vi "Get New Index.vi"(10 "last index":i32, 11 "control index":i32) -> (3 "new index":i32)   [LabVIEW 2015, in "LVJSON.lvlib" / "Index JSON Array.xnode"]
uses:
  Index JSON Array.xnode
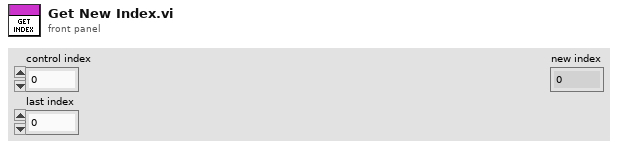
[diagram p1: front panel]
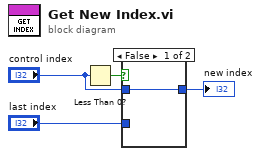
[diagram p0: block diagram]
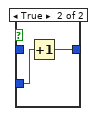
[diagram p2: hidden frame]
diagram:
  n1 = Less Than 0?(x="control index") -> (x < 0?=w4:bool)
  n2 = case shown="False" w4 {
    tunnel: [w5 w6] -> w2
    tunnel: "control index" -> [w5 _]
    tunnel: "last index" -> [_ w7]
    frame False {
    }
    frame True {
      n3 = Increment(x=w7) -> (x+1=w6:i32)
    }
  }
  "new index" <- w2
